vi "Simulation Record Get.vi"(8 "Error In":errorcluster, 11 "simulator":T12={"configuration"={"maxTime"=5.0, "enableVisualization"=TRUE, "Environment Definition"=path "iRobot Navigation State Machine.vi", "Record Location"=path "Simulation Record.xml", "autograde?"=TRUE, "interactive?"=FALSE, "Feedback Mode"=enum."debug navigation", "Robot State Charts"=[path "C:/Users/blueuser/Desktop/Robo Sim Berkley/cpsgrader-release-0.4/Simulators/EECS149lab/src/LabVIEW/statechart/Simulation Statechart.vi"], "statechart"=path "C:/Users/blueuser/Desktop/Robo Sim Berkley/cpsgrader-release-0.4/Simulators/EECS149lab/src/LabVIEW/statechart/Simulation Statechart.vi"}, "Statechart\ndisplay"=refnum, "first step?"=FALSE, "Robots Simulation Statecharts"=[], "Robots"=[]}) -> (0 "Error Out":errorcluster, 2 "record":T1={"configuration"={"maxTime"=5.0, "enableVisualization"=TRUE, "Environment Definition"=path "iRobot Navigation State Machine.vi", "Record Location"=path "Simulation Record.xml", "autograde?"=TRUE, "interactive?"=FALSE, "Feedback Mode"=enum."debug navigation", "Robot State Charts"=[path "C:/Users/blueuser/Desktop/Robo Sim Berkley/cpsgrader-release-0.4/Simulators/EECS149lab/src/LabVIEW/statechart/Simulation Statechart.vi"], "statechart"=path "C:/Users/blueuser/Desktop/Robo Sim Berkley/cpsgrader-release-0.4/Simulators/EECS149lab/src/LabVIEW/statechart/Simulation Statechart.vi"}, "trace"=[], "environment MD5"="", "statechart MD5"="", "record timestamp"=""} {"trace"."sensors"."Kobuki Sensors"."Charger Source" items=["DISCHARGING"=0, "DOCKING_CHARGED"=2, "DOCKING_CHARGING"=6, "ADAPTER_CHARGED"=18, "ADAPTER_CHARGING"=22]; "trace"."sensors"."accelerometer"."z axis (g)" format="%.3f"; "trace"."sensors"."accelerometer"."y axis (g)" format="%.3f"; "trace"."sensors"."accelerometer"."x axis (g)" format="%.3f"}, 3 "simulator":T12={"configuration"={"maxTime"=5.0, "enableVisualization"=TRUE, "Environment Definition"=path "iRobot Navigation State Machine.vi", "Record Location"=path "Simulation Record.xml", "autograde?"=TRUE, "interactive?"=FALSE, "Feedback Mode"=enum."debug navigation", "Robot State Charts"=[path "C:/Users/blueuser/Desktop/Robo Sim Berkley/cpsgrader-release-0.4/Simulators/EECS149lab/src/LabVIEW/statechart/Simulation Statechart.vi"], "statechart"=path "C:/Users/blueuser/Desktop/Robo Sim Berkley/cpsgrader-release-0.4/Simulators/EECS149lab/src/LabVIEW/statechart/Simulation Statechart.vi"}, "Statechart\ndisplay"=refnum, "first step?"=FALSE, "Robots Simulation Statecharts"=[], "Robots"=[]})   [LabVIEW 2015]
uses:
  Simulator.ctl
  CyberSim interface/Simulation Configuration.ctl
  autograder/feedbackMode.ctl
  Multi Bot Code/RobotData.ctl
  <instrlib>/DC Motor Controller/HAIOL/DC Motor Controller.lvclass
  Simulation Record.ctl
  Simulation Trace Element.ctl
  shared/Sensors.ctl
  shared/Accelerometer.ctl
  Kobuki/KobukiSensors.ctl
  Kobuki/Kobuki Bumps and WheelDrops.ctl
  Kobuki/Kobuki Buttons.ctl
  Simulated Position.ctl
  Simulated Orientation.ctl
  Simulation Trace Operation.ctl
panel:
  # "Electrical: charging, battery, OI mode"
  # "Sensors: bump, cliff, button, wheel drop"
  # "Motors:"
  # "Inertia"
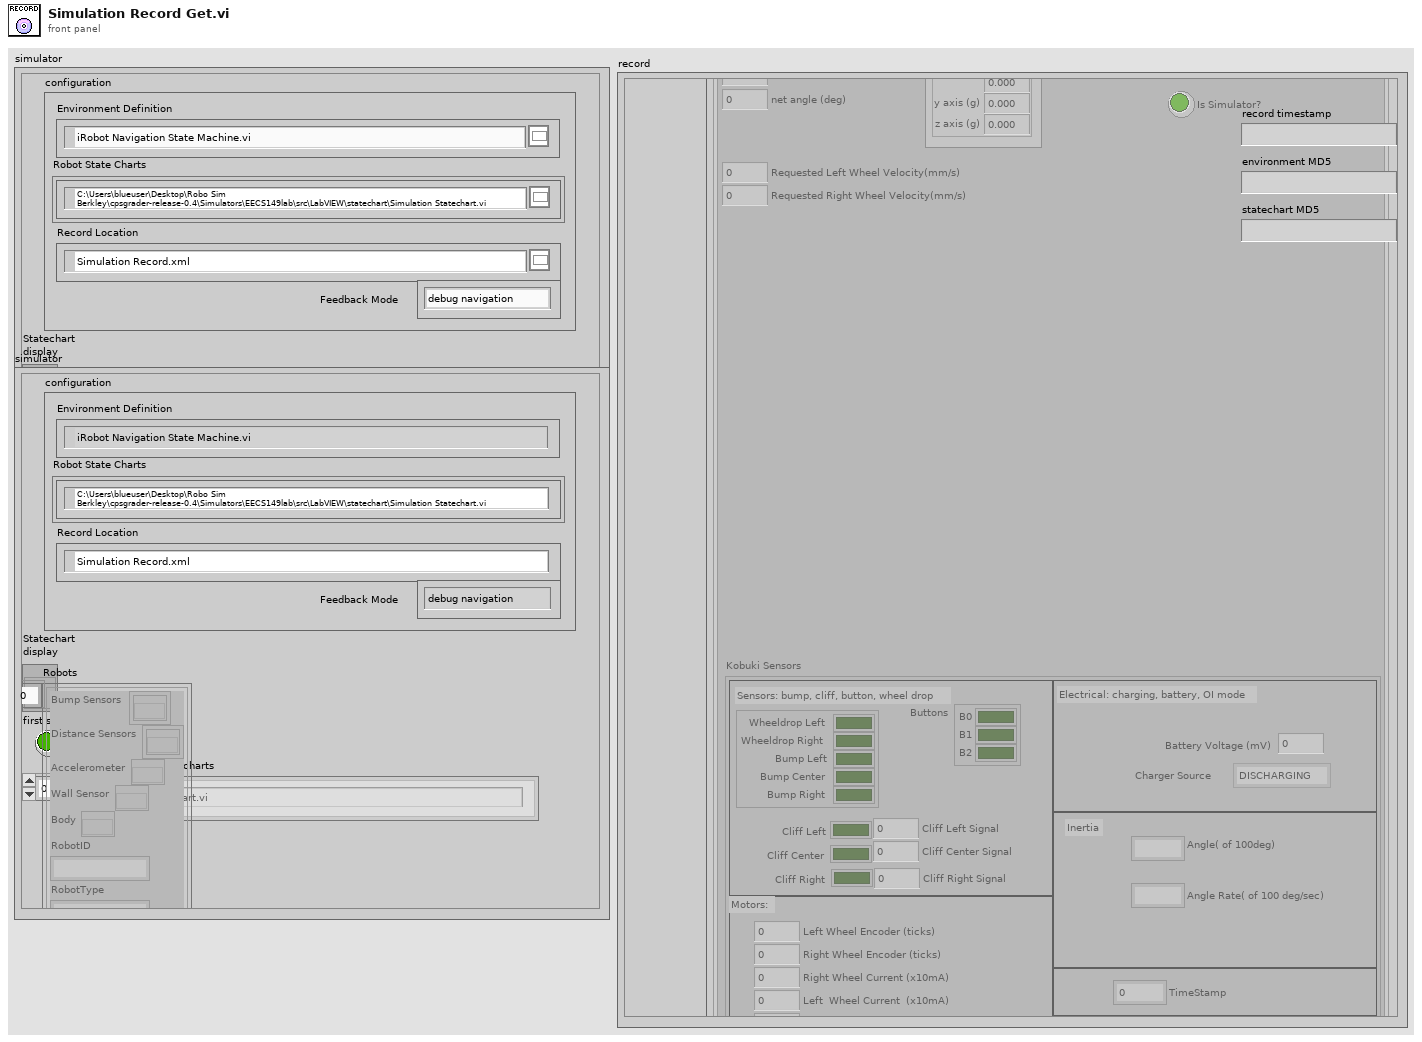
[diagram p1: front panel]
types:
  T1 = typedef "Simulation Record.ctl" = cluster{"configuration":T2, "trace":T4[], "environment MD5":string, "statechart MD5":string, "record timestamp":string}
  T2 = typedef "Simulation Configuration.ctl" = cluster{"maxTime":sgl, "enableVisualization":bool, "Environment Definition":path, "Record Location":path, "autograde?":bool, "interactive?":bool, "Feedback Mode":T3, "Robot State Charts":path[], "statechart":path}
  T3 = typedef "feedbackMode.ctl" = enum32{"debug navigation", "debug hill climb", "autograde navigation", "autograde hill climb"}
  T4 = typedef "Simulation Trace Element.ctl" = cluster{"sensors":T5, "position":T10, "orientation":T11, "Simulation Time (s)":sgl}
  T5 = typedef "Sensors.ctl" = cluster{"net distance (mm)":i32, "net angle (deg)":i32, "accelerometer":T6, "Is Simulator?":bool, "Kobuki Sensors":T7, "Requested Left Wheel Velocity(mm/s)":i32, "Requested Right Wheel Velocity(mm/s)":i32}
  T6 = typedef "Accelerometer.ctl" = cluster{"x axis (g)":dbl, "y axis (g)":dbl, "z axis (g)":dbl}
  T7 = typedef "KobukiSensors.ctl" = cluster{"Bumps + Wheel Drops":T8, "Cliff Left":bool, "Cliff Center":bool, "Cliff Right":bool, "Cliff Left Signal":u16, "Cliff Center Signal":u16, "Cliff Right Signal":u16, "Buttons":T9, "Left Wheel Encoder (ticks)":u16, "Right Wheel Encoder (ticks) ":u16, "Left  Wheel PWM":i8, "Right Wheel PWM":i8, "Left Wheel OverCurrent":bool, "Right Wheel OverCurrent ":bool, "Right Wheel Current (x10mA)":i16, "Left  Wheel Current  (x10mA)":i16, "TimeStamp":u16, "Battery Voltage (mV)":i16, "Angle( of 100deg)":i16, "Angle Rate( of 100 deg/sec)":i16, "Charger Source ":i8}
  T8 = typedef "Kobuki Bumps and WheelDrops.ctl" = cluster{"Wheeldrop Left":bool, "Wheeldrop Right":bool, "Bump Left":bool, "Bump Center":bool, "Bump Right":bool}
  T9 = typedef "Kobuki Buttons.ctl" = cluster{"B0":bool, "B1":bool, "B2":bool}
  T10 = typedef "Simulated Position.ctl" = cluster{"x (m)":sgl, "y (m)":sgl, "z (m)":sgl}
  T11 = typedef "Simulated Orientation.ctl" = cluster{"roll (deg)":sgl, "pitch (deg)":sgl, "yaw (deg)":sgl}
  T12 = typedef "Simulator.ctl" = cluster{"configuration":T2, "Statechart\ndisplay":refnum<vi>, "first step?":bool, "Robots Simulation Statecharts":path[], "Robots":T13[]}
  T13 = typedef "RobotData.ctl" = cluster{"Bump Sensors":refnum<k20>[], "Distance Sensors":refnum<k20>[], "Accelerometer":refnum<k20>, "Wall Sensor":refnum<k20>, "Body":refnum<k20>, "RobotID":string, "RobotType":string, "Left Motor":refnum<class "DC Motor Controller.lvclass">, "Right Motor":refnum<class "DC Motor Controller.lvclass">}
  T14 = typedef "Simulation Trace Operation.ctl" = enum16{"Initialize", "Record Trace Element", "Get Trace"}
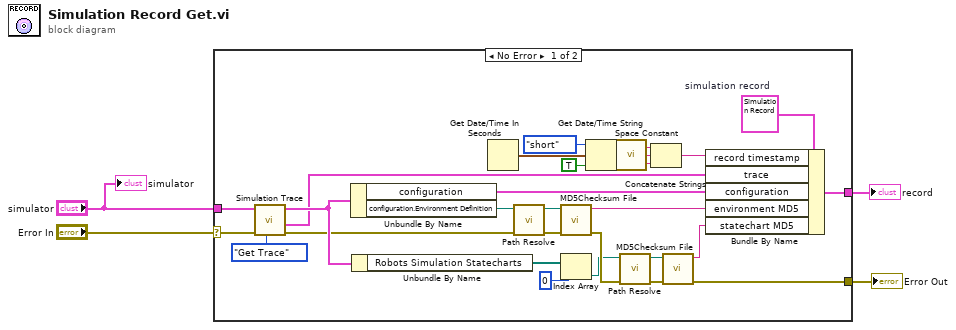
[diagram p0: block diagram]
diagram:
  n1 = case shown="No Error" "Error In" {
    selector: "Error In" -> [w8 w33]
    tunnel: [w32 w33] -> w4
    tunnel: "simulator" -> [w31 _]
    tunnel: [w30 _] -> w3
    frame No Error {
      w28 = T1 {"configuration"={"maxTime"=0.0, "enableVisualization"=FALSE, "Environment Definition"=path "", "Record Location"=path "", "autograde?"=FALSE, "interactive?"=FALSE, "Feedback Mode"=enum."debug navigation", "Robot State Charts"=[path "C:/Users/blueuser/Desktop/Robo Sim Berkley/cpsgrader-release-0.4/Simulators/EECS149lab/src/LabVIEW/statechart/Simulation Statechart.vi"], "statechart"=path "C:/Users/blueuser/Desktop/Robo Sim Berkley/cpsgrader-release-0.4/Simulators/EECS149lab/src/LabVIEW/statechart/Simulation Statechart.vi"}, "trace"=[], "environment MD5"="", "statechart MD5"="", "record timestamp"=""}  # simulation record
      n2 = call "Simulation Trace.vi"("operation"=Simulation_Trace_Operation."Get Trace", "error in"=w8, "simulator"=w31) -> ("error out"=w19:errorcluster, "trace"=w23:T4[], "simulator"=w29:T12)  [unwired: 5 in, 1 out]
      n3 = Unbundle By Name(w29) -> ("configuration"=w25:T2, "configuration.Environment Definition"=w20:path)
      n4 = Unbundle By Name(w29) -> ("Robots Simulation Statecharts"=w7:path[])
      n5 = Get Date/Time In Seconds() -> (seconds since 1Jan1904=w10:timestamp)
      n6 = call "Path Resolve.vi"("Error In"=w19, "absolute or relative path"=w20) -> ("Error Out"=w22:errorcluster, "resolved path"=w21:path)  [unwired: 8 in]
      n7 = call <vilib>:"MD5Checksum File.vi"("error in (no error)"=w22, "Path"=w21) -> ("error out"=w16:errorcluster, "MD5 message-digest"=w27:string)  [unwired: 8 in]
      n8 = Index Array(array=w7, index=0) -> (element=w5:path)
      n9 = Get Date/Time String(date format (0)=enum16{"short", "long", "abbreviated"}."short", seconds (now)=w10, want seconds? (F)=TRUE) -> (date string=w13:string, time string=w12:string)
      n10 = call <vilib>:"Space Constant.vi"() -> ("String"=w11:string)
      n11 = call "Path Resolve.vi"("Error In"=w16, "absolute or relative path"=w5) -> ("Error Out"=w17:errorcluster, "resolved path"=w18:path)  [unwired: 8 in]
      n12 = Concatenate Strings(w13, w11, w12) -> (w9:string)
      n13 = call <vilib>:"MD5Checksum File.vi"("error in (no error)"=w17, "Path"=w18) -> ("error out"=w32:errorcluster, "MD5 message-digest"=w26:string)  [unwired: 8 in]
      n14 = Bundle By Name(cluster=w28, "record timestamp"=w9, "trace"=w23, "configuration"=w25, "environment MD5"=w27, "statechart MD5"=w26) -> (w30:T1)
    }
    frame Error {
    }
  }
  "Error Out" <- w4
  "record" <- w3
  "simulator" <- "simulator"
